vi "MeasureEQE_ActiveX.vi"(6 "Skip?":bool, 8 "error in (no error)":errorcluster, 9 "Save data file path":string, 10 "Scan settings":T1={"J-V scan"=TRUE, "J-t scan"=FALSE, "Min voltage (V)"=0.0, "Max voltage (V)"=1.4, "Step (V)"=0.01, "Measurement delay (ms)"=10.0, "1st scan FB-SC"=TRUE, "Inverted structure"=FALSE, "Stabilisation time (s)"=0.0, "Stabilisation mode"=0, "Stabilisation value (V or A) "=0.0, "Step time (s)"=1.0, "Integration time"=0, "Repeat light scans"=FALSE, "Stabilisation in the dark?"=FALSE, "J-t Min (V)"=0.0, "J-t Max (V)"=1.4, "J-t Step (V)"=0.01, "Max. power stabilisation"=FALSE, "J-t 1st scan FB-SC"=TRUE, "J-t Inverted structure"=FALSE, "Max power tracking"=FALSE, "Vmp (V)"=0.7, "Total stabilisation time (s)"=100.0, "J-t best pixel only"=0, "Max power best pixel only"=0, "Vmp from J-V scan"=FALSE, "Intensity dependence"=FALSE, "P dep best pixel only"=0, "External quantum efficiency"=FALSE, "EQE best pixel only"=0, "WL min (nm)"=300.0, "WL max (nm)"=900.0, "WL step (nm)"=5.0, "Wait (ms)"=100.0, "No. of repeat scans"=2.0, "Only repeat for best pixel"=0, "Chopper Freq.  (Hz)"=90.0, "Time Constant (s)"=2.0, "Stabilisation time step (s)"=1.0, "Illumination conditions"=2, "Scan rate min (V/s)"=0.1, "Scan rate max (V/s)"=1.0, "No. of scan rate steps"=1.0, "Scan rate voltage step priority"=FALSE, "Scan rate measurement delay priority"=FALSE, "J-t Illumination conditions"=0, "White bias  (no. of suns)"=200.0, "Max P stab. Specific voltage"=FALSE} {"J-t Illumination conditions" items=["Light only", "Dark only", "Light then dark", "Dark then light"]; "No. of scan rate steps" min=1.0 step=1.0; "Illumination conditions" items=["Light only", "Dark only", "Light then dark", "Dark then light", "Light then dark then light", "Dark then light then dark"]; "Time Constant (s)" items=["0.003", "0.01", "0.03", "0.1", "0.3", "1", "3", "10", "30", "100"]; "Only repeat for best pixel" items=["only for best pixel", "for best 2 pixels", "for best 3 pixels", "for best 4 pixels", "for best 5 pixels", "for best 6 pixels", "for best 7 pixels", "for all pixels"]; "No. of repeat scans" min=1.0 step=1.0; "EQE best pixel only" items=["only the best pixel", "the best 2 pixel", "the best 3 pixel", "the best 4 pixel", "the best 5 pixel", "the best 6 pixel", "the best 7 pixel", "all pixels"]; "P dep best pixel only" items=["only the best pixel", "the best 2 pixels", "the best 3 pixels", "the best 4 pixels", "the best 5 pixels", "the best 6 pixels", "the best 7 pixels", "all pixels"]; "Max power best pixel only" items=["only the best pixel", "the best 2 pixels", "the best 3 pixels", "the best 4 pixels", "the best 5 pixels", "the best 6 pixels", "the best 7 pixels", "all pixels"]; "J-t best pixel only" items=["only the best pixel", "the best 2 pixels", "the best 3 pixels", "the best 4 pixels", "the best 5 pixels", "the best 6 pixels", "the best 7 pixels", "all pixels"]; "Integration time" items=["Fast", "Normal", "High Accuracy"]; "Stabilisation mode" items=["V", "I"]; "Measurement delay (ms)" min=10.0}) -> (0 "error out":errorcluster, 1 "Min WL (nm)":string, 2 "Max WL (nm)":string, 3 "EQE data file path":path)   [LabVIEW 2016]
uses:
  TypeDefs/Settings Boolean.ctl
  TypeDefs/Scan settings.ctl
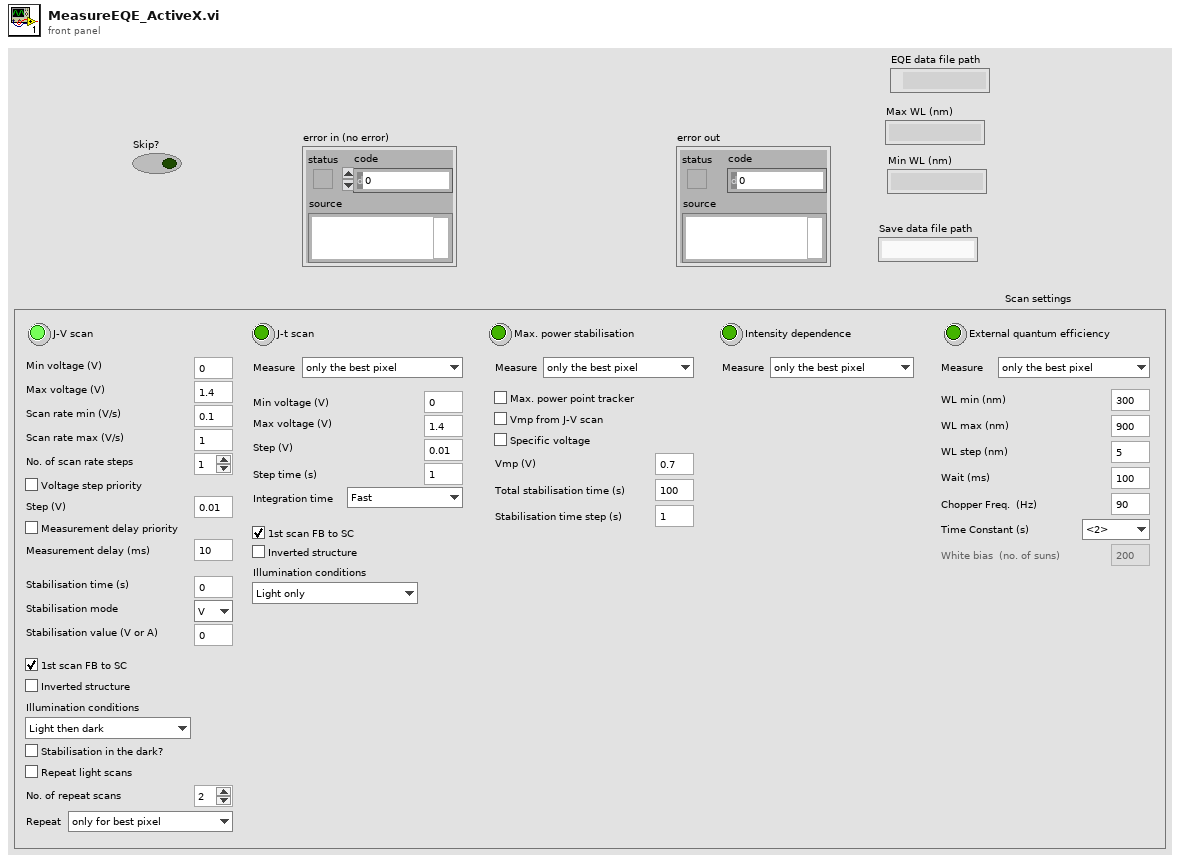
[diagram p1: front panel]
types:
  T1 = typedef "Scan settings.ctl" = cluster{"J-V scan":T2, "J-t scan":bool, "Min voltage (V)":dbl, "Max voltage (V)":dbl, "Step (V)":dbl, "Measurement delay (ms)":dbl, "1st scan FB-SC":bool, "Inverted structure":bool, "Stabilisation time (s)":dbl, "Stabilisation mode":u16, "Stabilisation value (V or A) ":dbl, "Step time (s)":dbl, "Integration time":u16, "Repeat light scans":bool, "Stabilisation in the dark?":bool, "J-t Min (V)":dbl, "J-t Max (V)":dbl, "J-t Step (V)":dbl, "Max. power stabilisation":bool, "J-t 1st scan FB-SC":bool, "J-t Inverted structure":bool, "Max power tracking":bool, "Vmp (V)":dbl, "Total stabilisation time (s)":dbl, "J-t best pixel only":u16, "Max power best pixel only":u16, "Vmp from J-V scan":bool, "Intensity dependence":bool, "P dep best pixel only":u16, "External quantum efficiency":bool, "EQE best pixel only":u16, "WL min (nm)":dbl, "WL max (nm)":dbl, "WL step (nm)":dbl, "Wait (ms)":dbl, "No. of repeat scans":dbl, "Only repeat for best pixel":u16, "Chopper Freq.  (Hz)":dbl, "Time Constant (s)":dbl, "Stabilisation time step (s)":dbl, "Illumination conditions":u16, "Scan rate min (V/s)":dbl, "Scan rate max (V/s)":dbl, "No. of scan rate steps":dbl, "Scan rate voltage step priority":bool, "Scan rate measurement delay priority":bool, "J-t Illumination conditions":u16, "White bias  (no. of suns)":dbl, "Max P stab. Specific voltage":bool}
  T2 = typedef "Settings Boolean.ctl" = bool
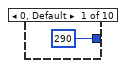
[diagram p2: hidden frame]
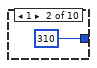
[diagram p3: hidden frame]
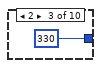
[diagram p4: hidden frame]
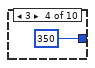
[diagram p5: hidden frame]
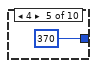
[diagram p6: hidden frame]
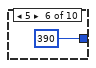
[diagram p7: hidden frame]
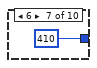
[diagram p8: hidden frame]
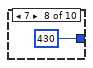
[diagram p9: hidden frame]
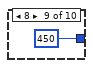
[diagram p10: hidden frame]
diagram:
  n1 = case shown="False" "Skip?" {
    tunnel: "error in (no error)" -> [w292 w304]
    tunnel: [w27 w304] -> w2
    frame False {
      w34 = 2000.0  # Buffer (ms)
      w35 = 11000.0  # Grating change time (ms)
      w38 = 2000.0  # Filter change time (ms)
      w39 = 22000.0  # initialisation time (ms)
      w42 = 1150.0  # time to change wl and measure (ms)
      # "Reduce min by one step"
      # "click \"Re-initialize to default value\""
      # "right-click \"Time constant\""
      # "click \"Clear graph\""
      # "click \"Ok\""
      # "Save file"
      # "click \"Save scan data\""
      # "click \"File\""
      # "click \"Take a simple wavelength scan\""
      # "click \"Scan\""
      # "Click \"OK\""
      # "Set wait"
      # "Set wavlength step"
      # "Set end wavlength"
      # "Set start wavlength"
      # "click \"Click Setup Scan Wavelength Parameters\""
      # "click \"Scan\""
      # "click \"OK\""
      # "click \"AC\""
      # "click \"Ref Type\""
      # "set chopper frequency (Hz)"
      # "choose time constant"
      # "click \"Time Constant\""
      # "click \"CHANNEL 2\""
      # "click \"Channel Setup\""
      # "click \"Setup Parameters\""
      # "click \"Detector\""
      n2 = Automation Open(error in (no error)=w292, Automation Refnum=refnum<k7> refnum ("AutoItX3Lib.IAutoItX3")) -> (Automation Refnum=w257:refnum<k7>, error out=w256:errorcluster)  [unwired: 2 in]
      n3 = invoke class="IAutoItX3" method="WinActivate"(reference=w257, error in=w256, "strTitle"="Newport Oriel Tracq Basic Version 6.2", "strText"="") -> (reference out=w291:refnum<k7>, error out=w284:errorcluster)  [unwired: 1 in, 3 out]
      n4 = invoke class="IAutoItX3" method="WinWaitActive"(reference=w291, error in=w284, "strTitle"="Newport Oriel Tracq Basic Version 6.2", "strText"="", "nTimeout"=2000) -> (reference out=w285:refnum<k7>, error out=w283:errorcluster)  [unwired: 1 in, 4 out]
      n5 = invoke class="IAutoItX3" method="MouseClick"(reference=w285, error in=w283, "strButton"="primary", "nX"=250, "nY"=40, "nClicks"=1) -> (reference out=w277:refnum<k7>, error out=w276:errorcluster)  [unwired: 2 in, 6 out]
      n6 = invoke class="IAutoItX3" method="Sleep"(reference=w277, error in=w276, "nMilliseconds"=100) -> (reference out=w271:refnum<k7>, error out=w270:errorcluster)  [unwired: 1 in, 2 out]
      n7 = invoke class="IAutoItX3" method="MouseClick"(reference=w271, error in=w270, "strButton"="primary", "nX"=290, "nY"=90, "nClicks"=1) -> (reference out=w266:refnum<k7>, error out=w265:errorcluster)  [unwired: 2 in, 6 out]
      n8 = invoke class="IAutoItX3" method="WinWaitActive"(reference=w266, error in=w265, "strTitle"="Merlin Setup", "strText"="", "nTimeout"=5000) -> (reference out=w251:refnum<k7>, error out=w250:errorcluster)  [unwired: 1 in, 4 out]
      n9 = invoke class="IAutoItX3" method="MouseClick"(reference=w251, error in=w250, "strButton"="primary", "nX"=450, "nY"=70, "nClicks"=1) -> (reference out=w242:refnum<k7>, error out=w241:errorcluster)  [unwired: 2 in, 6 out]
      n10 = invoke class="IAutoItX3" method="Sleep"(reference=w242, error in=w241, "nMilliseconds"=100) -> (reference out=w244:refnum<k7>, error out=w243:errorcluster)  [unwired: 1 in, 2 out]
      n11 = invoke class="IAutoItX3" method="MouseClick"(reference=w244, error in=w243, "strButton"="primary", "nX"=365, "nY"=140, "nClicks"=1) -> (reference out=w235:refnum<k7>, error out=w234:errorcluster)  [unwired: 2 in, 6 out]
      n12 = invoke class="IAutoItX3" method="Sleep"(reference=w235, error in=w234, "nMilliseconds"=100) -> (reference out=w19:refnum<k7>, error out=w18:errorcluster)  [unwired: 1 in, 2 out]
      n13 = Unbundle By Name("Scan settings") -> ("WL min (nm)"=w5:dbl, "WL max (nm)"=w33:dbl, "WL step (nm)"=w6:dbl, "Wait (ms)"=w32:dbl, "Chopper Freq.  (Hz)"=w51:dbl, "Time Constant (s)"=w54:dbl)
      n14 = invoke class="IAutoItX3" method="MouseClick"(reference=w19, error in=w18, "strButton"="secondary", "nX"=865, "nY"=295, "nClicks"=1) -> (reference out=w21:refnum<k7>, error out=w20:errorcluster)  [unwired: 2 in, 6 out]
      n15 = invoke class="IAutoItX3" method="Sleep"(reference=w21, error in=w20, "nMilliseconds"=100) -> (reference out=w10:refnum<k7>, error out=w9:errorcluster)  [unwired: 1 in, 2 out]
      n16 = case shown="9" w54 {
        tunnel: [290 310 330 350 370 390 410 430 450 470] -> w52
        frame 0, Default {
        }
        frame 1 {
        }
        frame 2 {
        }
        frame 3 {
        }
        frame 4 {
        }
        frame 5 {
        }
        frame 6 {
        }
        frame 7 {
        }
        frame 8 {
        }
        frame 9 {
        }
      }
      n17 = Subtract(x=w5, y=w6) -> (x-y=w4:dbl)
      n18 = invoke class="IAutoItX3" method="MouseClick"(reference=w10, error in=w9, "strButton"="primary", "nX"=900, "nY"=300, "nClicks"=1) -> (reference out=w12:refnum<k7>, error out=w11:errorcluster)  [unwired: 2 in, 6 out]
      n19 = Number To Fractional String(number=w33) -> (F-format string=w48:string)  [unwired: 3 in]
      "Max WL (nm)" <- w48
      n20 = Number To Fractional String(number=w6) -> (F-format string=w47:string)  [unwired: 3 in]
      n21 = Number To Fractional String(number=w32) -> (F-format string=w46:string)  [unwired: 3 in]
      n22 = Number To Fractional String(number=w51) -> (F-format string=w50:string)  [unwired: 3 in]
      n23 = Number To Fractional String(number=w4) -> (F-format string=w49:string)  [unwired: 3 in]
      "Min WL (nm)" <- w49
      n24 = invoke class="IAutoItX3" method="Sleep"(reference=w12, error in=w11, "nMilliseconds"=100) -> (reference out=w8:refnum<k7>, error out=w7:errorcluster)  [unwired: 1 in, 2 out]
      n25 = Subtract(x=w33, y=w4) -> (x-y=w45:dbl)
      n26 = Divide(x=w45, y=w6) -> (x/y=w44:dbl)
      n27 = Increment(x=w44) -> (x+1=w43:dbl)
      n28 = Add(x=w32, y=w42) -> (x+y=w41:dbl)
      n29 = Multiply(x=w43, y=w41) -> (x*y=w40:dbl)
      n30 = invoke class="IAutoItX3" method="MouseClick"(reference=w8, error in=w7, "strButton"="primary", "nX"=865, "nY"=310, "nClicks"=1) -> (reference out=w232:refnum<k7>, error out=w231:errorcluster)  [unwired: 2 in, 6 out]
      n31 = Multiply(x=w38, y=2.0) -> (x*y=w36:dbl)
      n32 = invoke class="IAutoItX3" method="Sleep"(reference=w232, error in=w231, "nMilliseconds"=100) -> (reference out=w225:refnum<k7>, error out=w224:errorcluster)  [unwired: 1 in, 2 out]
      n33 = Compound Arithmetic op=ADD(w40, w39, w36, w35, w34) -> (w31:dbl)
      n34 = invoke class="IAutoItX3" method="MouseClick"(reference=w225, error in=w224, "strButton"="primary", "nX"=865, "nY"=w52, "nClicks"=1) -> (reference out=w227:refnum<k7>, error out=w226:errorcluster)  [unwired: 2 in, 6 out]
      n35 = To Long Integer(number=w31) -> (32bit integer=w30:i32)
      n36 = invoke class="IAutoItX3" method="Sleep"(reference=w227, error in=w226, "nMilliseconds"=100) -> (reference out=w223:refnum<k7>, error out=w222:errorcluster)  [unwired: 1 in, 2 out]
      n37 = invoke class="IAutoItX3" method="MouseClickDrag"(reference=w223, error in=w222, "strButton"="primary", "nX1"=870 ("nX"), "nY1"=370 ("nY"), "nX2"=825 ("nClicks"), "nY2"=370 ("nClicks")) -> (reference out=w259:refnum<k7>, error out=w258:errorcluster)  [unwired: 2 in, 7 out]
      n38 = invoke class="IAutoItX3" method="Send"(reference=w259, error in=w258, "strSendText"=w50) -> (reference out=w214:refnum<k7>, error out=w213:errorcluster)  [unwired: 2 in, 3 out]
      n39 = invoke class="IAutoItX3" method="Sleep"(reference=w214, error in=w213, "nMilliseconds"=100) -> (reference out=w216:refnum<k7>, error out=w215:errorcluster)  [unwired: 1 in, 2 out]
      n40 = invoke class="IAutoItX3" method="MouseClick"(reference=w216, error in=w215, "strButton"="primary", "nX"=910, "nY"=695, "nClicks"=1) -> (reference out=w205:refnum<k7>, error out=w204:errorcluster)  [unwired: 2 in, 6 out]
      n41 = invoke class="IAutoItX3" method="Sleep"(reference=w205, error in=w204, "nMilliseconds"=100) -> (reference out=w207:refnum<k7>, error out=w206:errorcluster)  [unwired: 1 in, 2 out]
      n42 = invoke class="IAutoItX3" method="MouseClick"(reference=w207, error in=w206, "strButton"="primary", "nX"=830, "nY"=740, "nClicks"=1) -> (reference out=w196:refnum<k7>, error out=w195:errorcluster)  [unwired: 2 in, 6 out]
      n43 = invoke class="IAutoItX3" method="Sleep"(reference=w196, error in=w195, "nMilliseconds"=100) -> (reference out=w198:refnum<k7>, error out=w197:errorcluster)  [unwired: 1 in, 2 out]
      n44 = invoke class="IAutoItX3" method="MouseClick"(reference=w198, error in=w197, "strButton"="primary", "nX"=1125, "nY"=75, "nClicks"=1) -> (reference out=w191:refnum<k7>, error out=w190:errorcluster)  [unwired: 2 in, 6 out]
      n45 = invoke class="IAutoItX3" method="WinWaitActive"(reference=w191, error in=w190, "strTitle"="Newport Oriel Tracq Basic Version 6.2", "strText"="", "nTimeout"=10000) -> (reference out=w176:refnum<k7>, error out=w175:errorcluster)  [unwired: 1 in, 4 out]
      n46 = invoke class="IAutoItX3" method="MouseClick"(reference=w176, error in=w175, "strButton"="primary", "nX"=50, "nY"=35, "nClicks"=1) -> (reference out=w178:refnum<k7>, error out=w177:errorcluster)  [unwired: 2 in, 6 out]
      n47 = invoke class="IAutoItX3" method="Sleep"(reference=w178, error in=w177, "nMilliseconds"=100) -> (reference out=w180:refnum<k7>, error out=w179:errorcluster)  [unwired: 1 in, 2 out]
      n48 = invoke class="IAutoItX3" method="MouseClick"(reference=w180, error in=w179, "strButton"="primary", "nX"=45, "nY"=55, "nClicks"=1) -> (reference out=w171:refnum<k7>, error out=w170:errorcluster)  [unwired: 2 in, 6 out]
      n49 = invoke class="IAutoItX3" method="WinWaitActive"(reference=w171, error in=w170, "strTitle"="Enter Scan Parameters", "strText"="", "nTimeout"=2000) -> (reference out=w162:refnum<k7>, error out=w161:errorcluster)  [unwired: 1 in, 4 out]
      n50 = invoke class="IAutoItX3" method="MouseClickDrag"(reference=w162, error in=w161, "strButton"="primary", "nX1"=675 ("nX"), "nY1"=470 ("nY"), "nX2"=600 ("nClicks"), "nY2"=470 ("nClicks")) -> (reference out=w164:refnum<k7>, error out=w163:errorcluster)  [unwired: 2 in, 7 out]
      n51 = invoke class="IAutoItX3" method="Send"(reference=w164, error in=w163, "strSendText"=w49) -> (reference out=w153:refnum<k7>, error out=w152:errorcluster)  [unwired: 2 in, 3 out]
      n52 = invoke class="IAutoItX3" method="MouseClickDrag"(reference=w153, error in=w152, "strButton"="primary", "nX1"=675 ("nX"), "nY1"=515 ("nY"), "nX2"=600 ("nClicks"), "nY2"=515 ("nClicks")) -> (reference out=w155:refnum<k7>, error out=w154:errorcluster)  [unwired: 2 in, 7 out]
      n53 = invoke class="IAutoItX3" method="Send"(reference=w155, error in=w154, "strSendText"=w48) -> (reference out=w144:refnum<k7>, error out=w143:errorcluster)  [unwired: 2 in, 3 out]
      n54 = invoke class="IAutoItX3" method="MouseClickDrag"(reference=w144, error in=w143, "strButton"="primary", "nX1"=675 ("nX"), "nY1"=560 ("nY"), "nX2"=600 ("nClicks"), "nY2"=560 ("nClicks")) -> (reference out=w146:refnum<k7>, error out=w145:errorcluster)  [unwired: 2 in, 7 out]
      n55 = invoke class="IAutoItX3" method="Send"(reference=w146, error in=w145, "strSendText"=w47) -> (reference out=w135:refnum<k7>, error out=w134:errorcluster)  [unwired: 2 in, 3 out]
      n56 = invoke class="IAutoItX3" method="MouseClickDrag"(reference=w135, error in=w134, "strButton"="primary", "nX1"=675 ("nX"), "nY1"=600 ("nY"), "nX2"=600 ("nClicks"), "nY2"=600 ("nClicks")) -> (reference out=w137:refnum<k7>, error out=w136:errorcluster)  [unwired: 2 in, 7 out]
      n57 = invoke class="IAutoItX3" method="Send"(reference=w137, error in=w136, "strSendText"=w46) -> (reference out=w124:refnum<k7>, error out=w123:errorcluster)  [unwired: 2 in, 3 out]
      n58 = invoke class="IAutoItX3" method="MouseClick"(reference=w124, error in=w123, "strButton"="primary", "nX"=801, "nY"=425, "nClicks"=1) -> (reference out=w126:refnum<k7>, error out=w125:errorcluster)  [unwired: 2 in, 6 out]
      n59 = invoke class="IAutoItX3" method="WinWaitActive"(reference=w126, error in=w125, "strTitle"="Newport Oriel Tracq Basic Version 6.2", "strText"="", "nTimeout"=2000) -> (reference out=w115:refnum<k7>, error out=w114:errorcluster)  [unwired: 1 in, 4 out]
      n60 = invoke class="IAutoItX3" method="MouseClick"(reference=w115, error in=w114, "strButton"="primary", "nX"=50, "nY"=35, "nClicks"=1) -> (reference out=w117:refnum<k7>, error out=w116:errorcluster)  [unwired: 2 in, 6 out]
      n61 = invoke class="IAutoItX3" method="Sleep"(reference=w117, error in=w116, "nMilliseconds"=100) -> (reference out=w107:refnum<k7>, error out=w106:errorcluster)  [unwired: 1 in, 2 out]
      n62 = invoke class="IAutoItX3" method="MouseClick"(reference=w107, error in=w106, "strButton"="primary", "nX"=60, "nY"=80, "nClicks"=1) -> (reference out=w109:refnum<k7>, error out=w108:errorcluster)  [unwired: 2 in, 6 out]
      n63 = invoke class="IAutoItX3" method="Sleep"(reference=w109, error in=w108, "nMilliseconds"=w30) -> (reference out=w92:refnum<k7>, error out=w91:errorcluster)  [unwired: 1 in, 2 out]
      n64 = invoke class="IAutoItX3" method="MouseClick"(reference=w92, error in=w91, "strButton"="primary", "nX"=15, "nY"=35, "nClicks"=1) -> (reference out=w100:refnum<k7>, error out=w99:errorcluster)  [unwired: 2 in, 6 out]
      n65 = invoke class="IAutoItX3" method="Sleep"(reference=w100, error in=w99, "nMilliseconds"=100) -> (reference out=w94:refnum<k7>, error out=w93:errorcluster)  [unwired: 1 in, 2 out]
      n66 = invoke class="IAutoItX3" method="MouseClick"(reference=w94, error in=w93, "strButton"="primary", "nX"=30, "nY"=75, "nClicks"=1) -> (reference out=w87:refnum<k7>, error out=w86:errorcluster)  [unwired: 2 in, 6 out]
      n67 = invoke class="IAutoItX3" method="WinWaitActive"(reference=w87, error in=w86, "strTitle"="Choose file to write.", "strText"="", "nTimeout"=2000) -> (reference out=w76:refnum<k7>, error out=w75:errorcluster)  [unwired: 1 in, 4 out]
      n68 = String To Path(string="Save data file path") -> (path=→"EQE data file path":path)
      n69 = invoke class="IAutoItX3" method="Send"(reference=w76, error in=w75, "strSendText"="Save data file path") -> (reference out=w74:refnum<k7>, error out=w73:errorcluster)  [unwired: 2 in, 3 out]
      n70 = invoke class="IAutoItX3" method="MouseClick"(reference=w74, error in=w73, "strButton"="primary", "nX"=870, "nY"=670, "nClicks"=1) -> (reference out=w78:refnum<k7>, error out=w77:errorcluster)  [unwired: 2 in, 6 out]
      n71 = invoke class="IAutoItX3" method="WinWaitActive"(reference=w78, error in=w77, "strTitle"="Newport Oriel Tracq Basic Version 6.2", "strText"="", "nTimeout"=2000) -> (reference out=w68:refnum<k7>, error out=w67:errorcluster)  [unwired: 1 in, 4 out]
      n72 = invoke class="IAutoItX3" method="MouseClick"(reference=w68, error in=w67, "strButton"="primary", "nX"=1060, "nY"=115, "nClicks"=1) -> (reference out=w59:refnum<k7>, error out=w58:errorcluster)  [unwired: 2 in, 6 out]
      n73 = invoke class="IAutoItX3" method="WinActivate"(reference=w59, error in=w58, "strTitle"="Automated JV Measurement.vi", "strText"="") -> (reference out=w66:refnum<k7>, error out=w60:errorcluster)  [unwired: 1 in, 3 out]
      n74 = invoke class="IAutoItX3" method="WinWaitActive"(reference=w66, error in=w60, "strTitle"="Automated JV Measurement.vi", "strText"="", "nTimeout"=2000) -> (reference out=w57:refnum<k7>, error out=w56:errorcluster)  [unwired: 1 in, 4 out]
      n75 = Close Reference(reference=w57, error in (no error)=w56) -> (error out=w27:errorcluster)
    }
    frame True {
    }
  }
  "error out" <- w2
